vi "Read XML Tag.vi"(0 "XML String":string, 1 "ignore case? (F)":bool, 5 "Tag":string, 11 "error in (no error)":errorcluster) -> (4 "XML Tag Contents":string, 6 "Found":bool, 8 "String Bounds of Match":T1, 15 "error out":errorcluster)   [LabVIEW 2017, in "CL_G3_VIComponentBuilder.lvlib"]
doc: "Read out the XML Tag Contents for the given Tag in XML String"
uses:
  CL_G3_VIComponentBuilder.lvlib
  <vilib>/regexp/Match Regular Expression.xnode
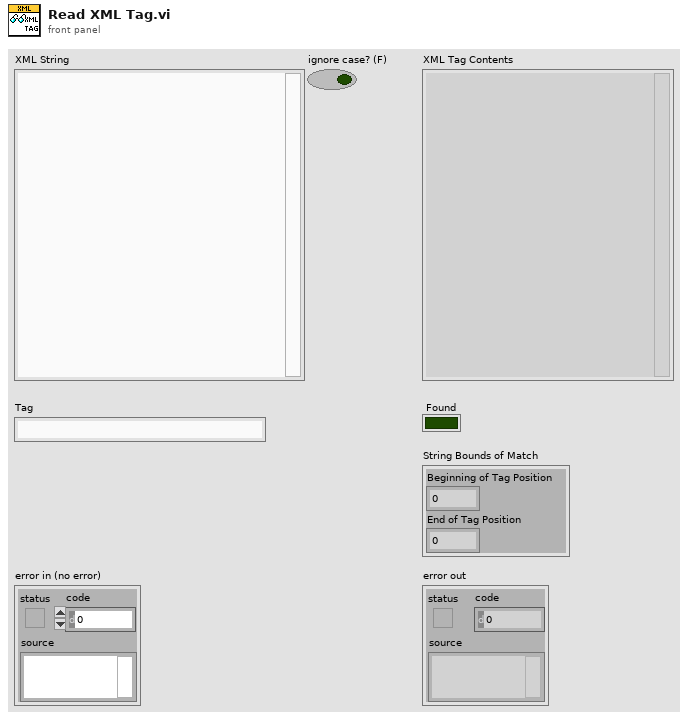
[diagram p1: front panel]
types:
  T1 = cluster{"Beginning of Tag Position":i32, "End of Tag Position":i32}
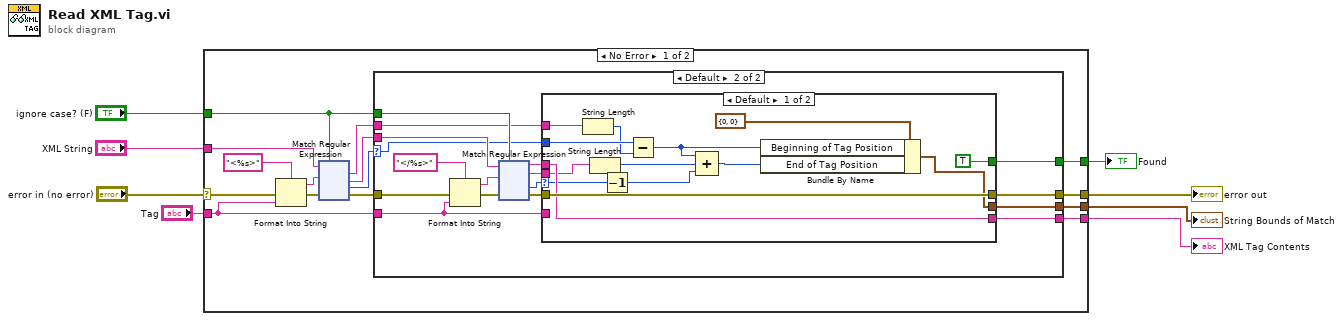
[diagram p0: block diagram]
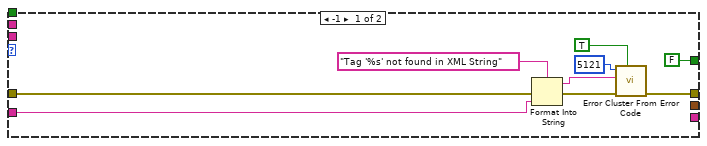
[diagram p2: hidden frame]
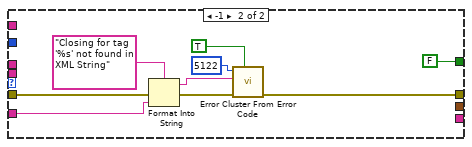
[diagram p3: hidden frame]
diagram:
  n1 = case shown="No Error" "error in (no error)" {
    selector: "error in (no error)" -> [w18 w301]
    tunnel: [w15 w301] -> w8
    tunnel: "Tag" -> [w12 _]
    tunnel: "ignore case? (F)" -> [w17 _]
    tunnel: "XML String" -> [w16 _]
    tunnel: [w14 _] -> w3
    tunnel: [w11 _] -> w2
    tunnel: [w9 _] -> w1
    frame No Error {
      n2 = Format Into String(format string="<%s>", error in=w18, w12) -> (resulting string=w21:string, error out=w20:errorcluster)  [unwired: 1 in]
      n3 = xnode "Match Regular Expression"("input string"=w16, "regular expression"=w21, "error in"=w20, "ignore case? (F)"=w17) -> ("whole match"=w10:string, "after match"=w22:string, "offset past match"=w13:i32, "error out"=w19:errorcluster)  [unwired: 2 in, 1 out]
      n4 = case shown="Default" w13 {
        selector: w13 -> [_ w36]
        tunnel: w22 -> [_ w48]
        tunnel: w19 -> [w32 w46]
        tunnel: w17 -> [_ w44]
        tunnel: [w27 w41] -> w15
        tunnel: [_ w39] -> w14
        tunnel: w12 -> [w31 w38]
        tunnel: [FALSE w37] -> w11
        tunnel: w10 -> [_ w35]
        tunnel: [_ w34] -> w9
        frame -1 {
          n5 = Format Into String(format string="Tag '%s' not found in XML String", error in=w32, w31) -> (resulting string=w26:string, error out=w28:errorcluster)  [unwired: 1 in]
          n6 = call <vilib>:"Error Cluster From Error Code.vi"("show call chain? (False)"=TRUE, "error in (no error)"=w28, "error message (\"\")"=w26, "error code (0)"=5121 ("Error Code")) -> ("error out"=w27:errorcluster)  [unwired: 5 in]
        }
        frame Default {
          n7 = Format Into String(format string="</%s>", error in=w46, w38) -> (resulting string=w47:string, error out=w45:errorcluster)  [unwired: 1 in]
          n8 = xnode "Match Regular Expression"("input string"=w48, "regular expression"=w47, "error in"=w45, "ignore case? (F)"=w44) -> ("before match"=w40:string, "whole match"=w33:string, "offset past match"=w42:i32, "error out"=w43:errorcluster)  [unwired: 2 in, 1 out]
          n9 = case shown="Default" w42 {
            selector: w42 -> [w52 _]
            tunnel: w43 -> [w63 w72]
            tunnel: [w63 w68] -> w41
            tunnel: w40 -> [w56 _]
            tunnel: [w56 _] -> w39
            tunnel: w38 -> [_ w71]
            tunnel: [TRUE FALSE] -> w37
            tunnel: w36 -> [w60 _]
            tunnel: w35 -> [w61 _]
            tunnel: [w57 _] -> w34
            tunnel: w33 -> [w53 _]
            frame Default {
              n10 = String Length(string=w61) -> (length=w59:i32)
              n11 = String Length(string=w53) -> (length=w51:i32)
              n12 = Decrement(x=w52) -> (x-1=w50:i32)
              n13 = Subtract(x=w60, y=w59) -> (x-y=w55:i32)
              n14 = Compound Arithmetic op=ADD(w55, w51, w50) -> (w54:i32)
              n15 = Bundle By Name(cluster=T1 {"Beginning of Tag Position"=0, "End of Tag Position"=0}, "Beginning of Tag Position"=w55, "End of Tag Position"=w54) -> (w57:T1)
            }
            frame -1 {
              n16 = Format Into String(format string="Closing for tag '%s' not found in XML String", error in=w72, w71) -> (resulting string=w67:string, error out=w69:errorcluster)  [unwired: 1 in]
              n17 = call <vilib>:"Error Cluster From Error Code.vi"("show call chain? (False)"=TRUE, "error in (no error)"=w69, "error message (\"\")"=w67, "error code (0)"=5122 ("Error Code")) -> ("error out"=w68:errorcluster)  [unwired: 5 in]
            }
          }
        }
      }
    }
    frame Error {
    }
  }
  "XML Tag Contents" <- w3
  "error out" <- w8
  "Found" <- w2
  "String Bounds of Match" <- w1
